vi "StringToNativePath.vi"(1 "Agnostic Path":string) -> (0 "Native Path":path)   [LabVIEW 2017]
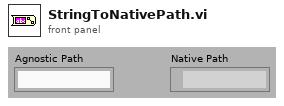
[diagram p1: front panel]
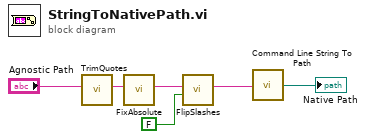
[diagram p0: block diagram]
diagram:
  n1 = call <vilib>:"TrimQuotes.vi"("With \""="Agnostic Path") -> ("Without \""=w4:string)  [unwired: 10 in]
  n2 = call <vilib>:"FixAbsolute.vi"("Relative"=w4) -> ("Absolute"=w3:string)  [unwired: 10 in]
  n3 = call <vilib>:"FlipSlashes.vi"("ConfigFormat"=FALSE, "Before"=w3) -> ("After"=w2:string)  [unwired: 9 in]
  n4 = call <vilib>:"Command Line String To Path.vi"("string"=w2) -> ("path"=→"Native Path":path)
